vi "Remove Character.vi"(9 "Character to Remove":string="-", 10 "String":string) -> (1 "String Result":string, 2 "Array Result":string[](array[string]))   [LabVIEW 2016]
panel:
  out "Array - String":string[](array[string])
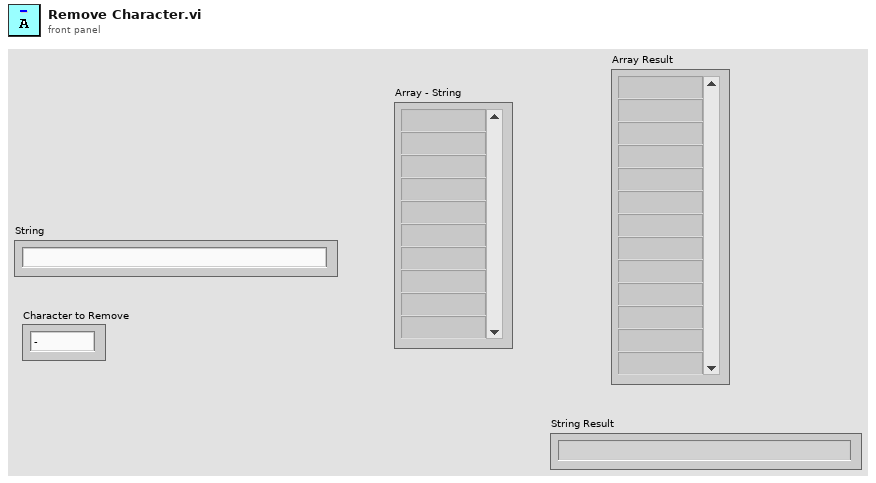
[diagram p1: front panel]
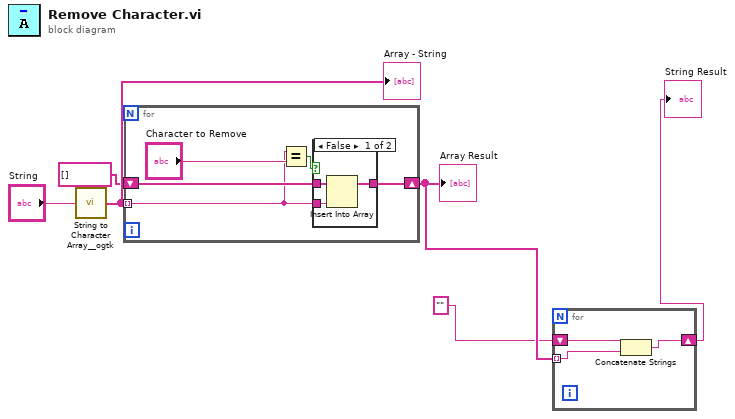
[diagram p0: block diagram]
diagram:
  n1 = call <userlib>:"String to Character Array__ogtk.vi"("Input String"="String") -> ("Character Array"=w5:string[])
  "Array - String" <- w5
  n2 = for {
    tunnel: w5 -> [w7] mode=indexing
    shift-right: [w9] -> w3
    shift-left: string[] [] ("Character Array") -> [w8]
    n3 = Equal?(x=w7, y="Character to Remove") -> (x = y?=w10:bool)
    n4 = case shown="False" w10 {
      tunnel: [w12 w15] -> w9
      tunnel: w8 -> [w14 w15]
      tunnel: w7 -> [w13 _]
      frame False {
        n5 = Insert Into Array(array=w14, new element=w13) -> (w12:string[])  [unwired: 1 in]
      }
      frame True {
      }
    }
  }
  "Array Result" <- w3
  n6 = for {
    tunnel: w3 -> [w17] mode=indexing
    shift-right: [w16] -> w1
    shift-left: "" ("delimiter (Tab)") -> [w18]
    n7 = Concatenate Strings(w18, w17) -> (w16:string)
  }
  "String Result" <- w1
